vi "Camera Tester.vi"() -> ()   [LabVIEW 2015]
uses:
  Left Variables.vi
panel:
  out "L Raw RB Y Center":u16
  out "L Raw RB X Center":u16
  out "L Raw LB Y Center":u16
  out "L Raw LB X Center":u16
  in  "STOP":bool
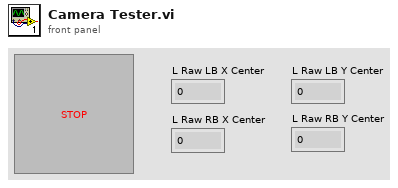
[diagram p1: front panel]
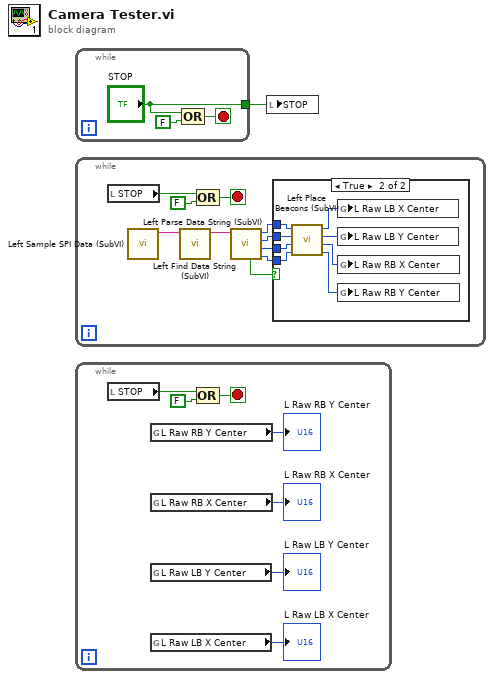
[diagram p0: block diagram]
diagram:
  n1 = while {
    tunnel: ["STOP"] -> w1
    stop <- w3 stop-if-true
    n2 = Compound Arithmetic op=OR("STOP", FALSE) -> (w3:bool)
  }
  n3 = while {
    stop <- w10 stop-if-true
    n4 = local read "STOP"() -> (w12:bool)
    n5 = call "Left Sample SPI Data (SubVI).vi"() -> ("Sampled Data"=w14:string)  [unwired: 11 in]
    n6 = call "Left Find Data String (SubVI).vi"("Sampled Data"=w14) -> ("Data String"=w13:string)  [unwired: 10 in]
    n7 = Compound Arithmetic op=OR(w12, FALSE) -> (w10:bool)
    n8 = call "Left Parse Data String (SubVI).vi"("Data String"=w13) -> ("o2 Y Center"=w5:u16, "o2 X Center"=w6:u16, "o1 Y Center"=w7:u16, "o1 X Center"=w8:u16, "Data Valid?"=w9:bool)  [unwired: 6 in]
    n9 = case shown="True" w9 {
      tunnel: w8 -> [_ w22]
      tunnel: w7 -> [_ w21]
      tunnel: w6 -> [_ w20]
      tunnel: w5 -> [_ w19]
      frame False {
      }
      frame True {
        n10 = call "Left Place Beacons (SubVI).vi"("o2 Y Center"=w19, "o2 X Center"=w20, "o1 Y Center"=w21, "o1 X Center"=w22) -> ("Raw RB Y Center"=w15:u16, "Raw RB X Center"=w16:u16, "Raw LB Y Center"=w17:u16, "Raw LB X Center"=w18:u16)  [unwired: 4 in]
        n11 = global write "Left Variables.vi" "L Raw LB X Center"(w18) -> ()
        n12 = global write "Left Variables.vi" "L Raw LB Y Center"(w17) -> ()
        n13 = global write "Left Variables.vi" "L Raw RB X Center"(w16) -> ()
        n14 = global write "Left Variables.vi" "L Raw RB Y Center"(w15) -> ()
      }
    }
  }
  n15 = while {
    stop <- w24 stop-if-true
    n16 = local read "STOP"() -> (w23:bool)
    n17 = global read "Left Variables.vi" "L Raw RB Y Center"() -> (→"L Raw RB Y Center":u16)
    n18 = global read "Left Variables.vi" "L Raw RB X Center"() -> (→"L Raw RB X Center":u16)
    n19 = global read "Left Variables.vi" "L Raw LB Y Center"() -> (→"L Raw LB Y Center":u16)
    n20 = global read "Left Variables.vi" "L Raw LB X Center"() -> (→"L Raw LB X Center":u16)
    n21 = Compound Arithmetic op=OR(w23, FALSE) -> (w24:bool)
  }
  n22 = local write "STOP"(w1) -> ()
